vi "GetColorCatchIndex.vi"(9 "Catch Color":dbl[](array[numeric]), 11 "Color":dbl) -> (2 "Catch Color Index":i16)   [LabVIEW 2018]
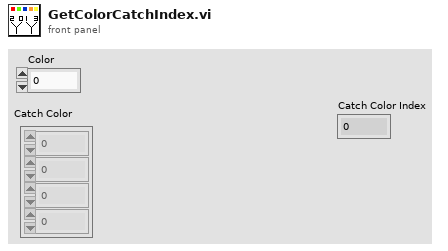
[diagram p1: front panel]
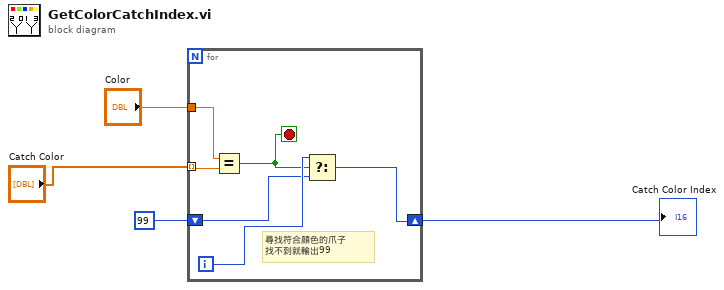
[diagram p0: block diagram]
diagram:
  n1 = for {
    tunnel: "Catch Color" -> [w10] mode=indexing
    shift-right: [w6] -> w2
    shift-left: 99 -> [w8]
    tunnel: "Color" -> [w5]
    i -> [w9]
    stop <- w7 stop-if-true
    # "尋找符合顏色的爪子\n找不到就輸出99"
    n2 = Equal?(x=w5, y=w10) -> (x = y?=w7:bool)
    n3 = Select(t=w9, s=w7, f=w8) -> (s? t:f=w6:i32)
  }
  "Catch Color Index" <- w2
